vi "Remove Device.vi"(8 "error in (no error)":errorcluster, 11 "Configuration UI in":refnum<class "Configuration UI.lvclass">) -> (0 "error out":errorcluster, 3 "Configuration UI out":refnum<class "Configuration UI.lvclass">)   [LabVIEW 2023, in "Configuration UI.lvlib" / "Configuration UI.lvclass"]
doc: "This routine:\n1. Deletes the instrument record by calling <b>Config:Delete Instrument Record</b>\n2. Refreshes the display by calling <b>Refresh Display</b>"
uses:
  Project/Configuration UI.lvclass
  Project/Configuration UI.lvclass/Configuration UI.ctl
  builds/Tools/Config.lvlibp/Config.lvclass
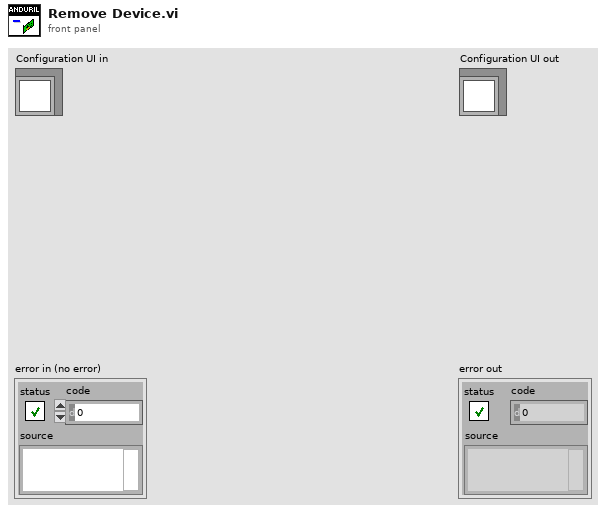
[diagram p1: front panel]
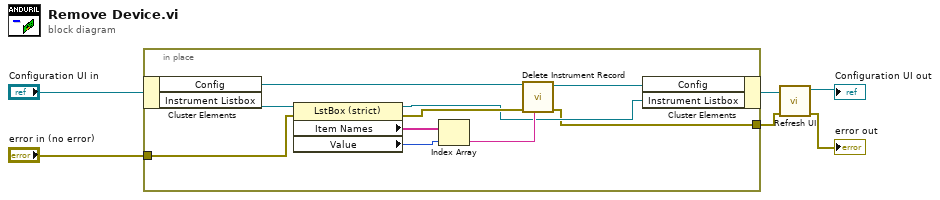
[diagram p0: block diagram]
diagram:
  n1 = in-place {
    in-place-border: [w8] -> w2
    in-place-border: "error in (no error)" -> [w7]
    n2 = in-place-cluster #1("Configuration UI in") -> ("Config"=w16:refnum<class "Config.lvclass">, "Instrument Listbox"=w14:refnum<vi>)
    n3 = property class="LstBox (strict)"(reference=w14, error in=w7) -> (reference out=w9:refnum<vi>, error out=w10:errorcluster, "Item Names"=w13:string[], "Value"=w12:i32)
    n4 = Index Array(array=w13, index=w12) -> (element=w11:string)
    n5 = call "Delete Instrument Record.vi"("Device"=w11, "error in"=w10, "Config in"=w16) -> ("error out"=w8:errorcluster, "Config out"=w15:refnum<class "Config.lvclass">)  [unwired: 7 in]
    n6 = in-place-cluster #1("Config"=w15, "Instrument Listbox"=w9) -> (w4:refnum<class "Configuration UI.lvclass">)
  }
  n7 = call "Refresh UI.vi"("error in (no error)"=w2, "Configuration UI in"=w4) -> ("error out"=→"error out":errorcluster, "Configuration UI out"=→"Configuration UI out":refnum<class "Configuration UI.lvclass">)  [unwired: 8 in]
